vi "Read Mutation Delta.vi"(8 "error in (no error)":errorcluster, 11 "Real Mutator in":refnum<class "Real Mutator.lvclass">) -> (0 "error out":errorcluster, 2 "Mutation Delta":cluster{"Upper":dbl, "Lower":dbl}, 3 "Real Mutator out":refnum<class "Real Mutator.lvclass">)   [LabVIEW 2016, in "Real Mutator.lvclass"]
uses:
  Real Mutator.lvclass
  Real Mutator.lvclass/Real Mutator.ctl
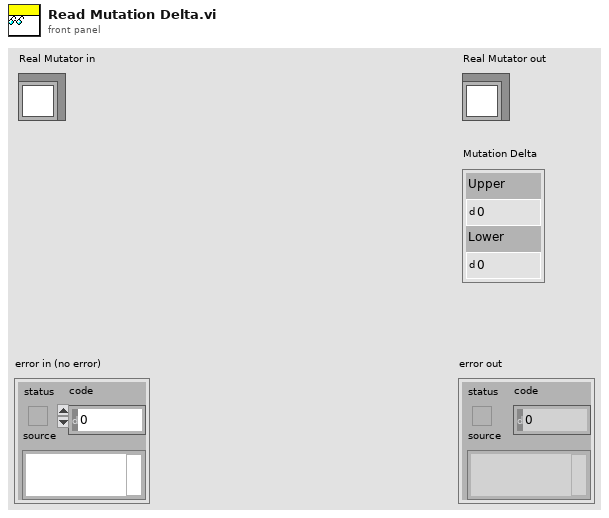
[diagram p1: front panel]
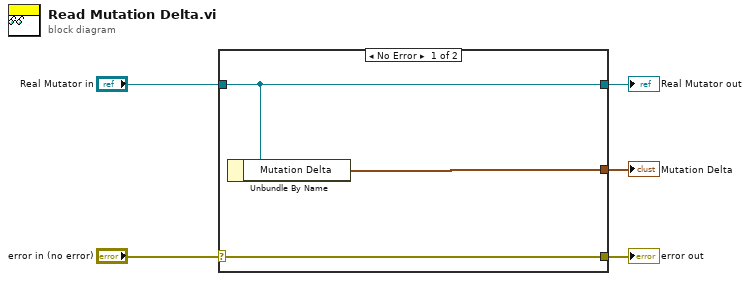
[diagram p0: block diagram]
diagram:
  n1 = case shown="No Error" "error in (no error)" {
    selector: "error in (no error)" -> [w8 w9]
    tunnel: [w8 w9] -> w4
    tunnel: [w7 w10] -> w2
    tunnel: "Real Mutator in" -> [w7 w10]
    tunnel: [w6 _] -> w1
    frame No Error {
      n2 = Unbundle By Name(w7) -> ("Mutation Delta"=w6:cluster{"Upper (1)":dbl, "Lower (-1)":dbl})
    }
    frame Error {
    }
  }
  "error out" <- w4
  "Real Mutator out" <- w2
  "Mutation Delta" <- w1
